vi "QWavelength.vi"(8 "error in (no error)":errorcluster, 11 "VISA resource name":refnum<visa-resource-name>) -> (0 "error out":errorcluster, 2 "Wavelength":dbl[unit], 3 "VISA resource name out":refnum<visa-resource-name>)   [LabVIEW 2013, in "Newport 1830-C.lvlib"]
doc: "Returns current wavelength setting"
uses:
  Newport 1830-C.lvlib
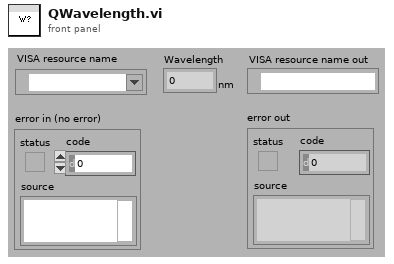
[diagram p1: front panel]
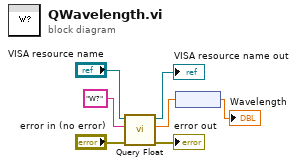
[diagram p0: block diagram]
diagram:
  n1 = call "Query Float.vi"("error in (no error)"="error in (no error)", "write buffer"="W?" ("command"), "VISA resource name In"="VISA resource name") -> ("error out"=→"error out":errorcluster, "float"=w2:dbl, "VISA resource name out"=→"VISA resource name out":refnum<visa-resource-name>)  [unwired: 6 in]
  n2 = node(w2) -> (→"Wavelength":dbl[unit])
